vi "Cycle Engine State.vi"(11 "Data":string) -> (3 "Cycle Engine State":string)   [LabVIEW 2016, in "GEA2_Toolkit.lvlib"]
uses:
  library/GEA2_Toolkit.lvlib
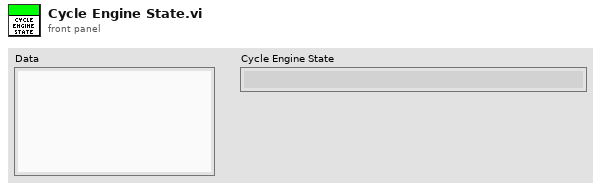
[diagram p1: front panel]
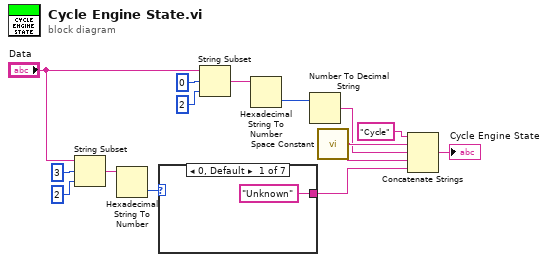
[diagram p0: block diagram]
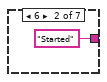
[diagram p2: hidden frame]
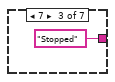
[diagram p3: hidden frame]
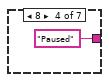
[diagram p4: hidden frame]
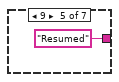
[diagram p5: hidden frame]
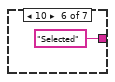
[diagram p6: hidden frame]
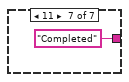
[diagram p7: hidden frame]
diagram:
  n1 = String Subset(string="Data", offset (0)=3, length (rest)=2 ("length (rest)")) -> (substring=w8:string)
  n2 = Hexadecimal String To Number(string=w8) -> (number=w10:u32)  [unwired: 2 in, 1 out]
  n3 = case shown="0, Default" w10 {
    tunnel: ["Unknown" "Started" "Stopped" "Paused" "Resumed" "Selected" "Completed"] -> w9
    frame 0, Default {
    }
    frame 6 {
    }
    frame 7 {
    }
    frame 8 {
    }
    frame 9 {
    }
    frame 10 {
    }
    frame 11 {
    }
  }
  n4 = String Subset(string="Data", offset (0)=0, length (rest)=2 ("length (rest)")) -> (substring=w5:string)
  n5 = Hexadecimal String To Number(string=w5) -> (number=w6:u32)  [unwired: 2 in, 1 out]
  n6 = Number To Decimal String(number=w6) -> (decimal integer string=w7:string)  [unwired: 1 in]
  n7 = call <vilib>:"Space Constant.vi"() -> ("String"=w11:string)
  n8 = Concatenate Strings("Cycle" ("string"), w11, w7, w11, w9) -> (→"Cycle Engine State":string)
